vi "Test UI.vi"() -> ()   [LabVIEW 2017]
panel:
  in  "Boolean":bool
  in  "Numeric":dbl
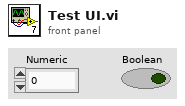
[diagram p1: front panel]
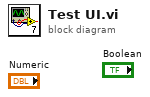
[diagram p0: block diagram]
diagram:
